vi "Global - Occurrence Loop Stop.vi"() -> ()   [LabVIEW 2023]
doc: "Global Variable that is used to stop parallel loops in the Simple Occurrence example."
panel:
  in  "Loop Stop":bool
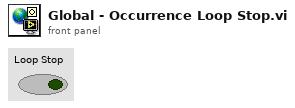
[diagram p1: front panel]
diagram:
